vi "Element by Index.vi"(8 "error in (no error)":errorcluster, 9 "Index":i32, 11 "Config Manager in":refnum<class "Config Manager.lvclass">) -> (0 "error out":errorcluster, 2 "Element":refnum<class "Config Element.lvclass">, 3 "Config Manager out":refnum<class "Config Manager.lvclass">)   [LabVIEW 2020, in "CDM-Config.lvlib" / "Config Manager.lvclass"]
uses:
  Config Manager.lvclass
  Config Element/Config Element.lvclass
  Config Manager.lvclass/Config Manager.ctl
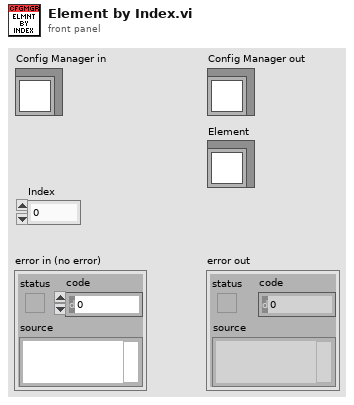
[diagram p1: front panel]
types:
  T1 = typedef "CDM-Config.lvlib/Config Manager.lvclass/Ref Data.ctl" = cluster{"Elements":refnum<class "Config Element.lvclass">[], "Hierarchy Map":map{string[], i32}, "Meta Name Map":map{string, i32[]}, "Element Map":map{refnum<class "Config Element.lvclass">, i32}, "Changed":bool[]}
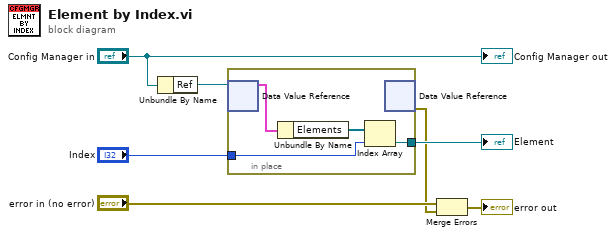
[diagram p0: block diagram]
diagram:
  n1 = Unbundle By Name("Config Manager in") -> ("Ref"=w6:refnum<data-value>)
  n2 = in-place {
    in-place-border: [w9] -> w4
    in-place-border: "Index" -> [w8]
    n3 = in-place-dvr #1(w6) -> (w11:T1)  [unwired: 1 out]
    n4 = Unbundle By Name(w11) -> ("Elements"=w10:refnum<class "Config Element.lvclass">[])
    n5 = Index Array(array=w10, index=w8) -> (element=w9:refnum<class "Config Element.lvclass">)
    n6 = in-place-dvr #1() -> (w1:errorcluster)  [unwired: 1 in, 1 out]
  }
  "Element" <- w4
  n7 = Merge Errors("error in (no error)", w1) -> (→"error out":errorcluster)
  "Config Manager out" <- "Config Manager in"
